vi "Konvolucio MCAN120803 Example_0003 ConnectBySerialNumber.vi"() -> ()   [LabVIEW 2011]
uses:
  <instrlib>/Konvolucio MCAN120803/Types/AdapterItemType.ctl
  C:/Program Files/National Instruments/LabVIEW 2011/instr.lib/Konvolucio MCAN120803/Private/Konvolucio.MCAN120803.API.dll
  Private/Konvolucio.MCAN120803.API.dll
  <instrlib>/Konvolucio MCAN120803/Public/Attributes/AttrGetSerialNumber.vi
  <instrlib>/Konvolucio MCAN120803/Konvolucio MCAN120803.lvlib
panel:
  out "Connected To:":string
  out "AdaptersOut":T1[](array[typedef])
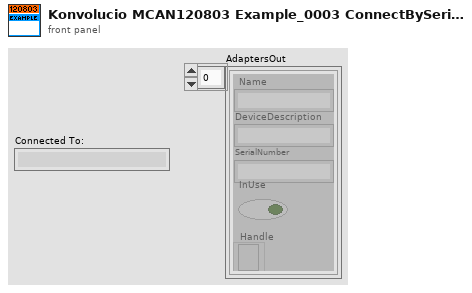
[diagram p1: front panel]
types:
  T1 = typedef "Konvolucio MCAN120803.lvlib/AdapterItemType.ctl" = cluster{"Name":string, "DeviceDescription":string, "SerialNumber":string, "InUse":bool, "Handle":refnum<k24>}
  T2 = typedef "Konvolucio MCAN120803.lvlib/CanHandleType.ctl" = cluster{"AdapterDevice":refnum<k24>}
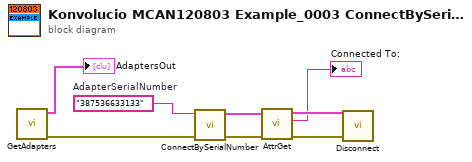
[diagram p0: block diagram]
diagram:
  w7 = "387536633133"  # AdapterSerialNumber
  n1 = call <instrlib>:"GetAdapters.vi"() -> ("error out"=w6:errorcluster, "AdaptersOut"=→"AdaptersOut":T1[])  [unwired: 10 in]
  n2 = call <instrlib>:"ConnectBySerialNumber.vi"("error in"=w6, "AdapterSerialNumber"=w7) -> ("error out"=w4:errorcluster, "CanHandleOut"=w3:T2)  [unwired: 8 in]
  n3 = call-poly <instrlib>:"AttrGet.vi"("error in"=w4, "CanHandleIn"=w3) -> ("error out"=w5:errorcluster, "Value"=→"Connected To:":string, "CanHandleOut"=w2:T2)  [unwired: 7 in]
  n4 = call <instrlib>:"Disconnect.vi"("error in"=w5, "CanHandleIn"=w2) -> ()  [unwired: 9 in, 1 out]
